vi "ClosestString.vi"(8 "array of frequencies":dbl[](array[numeric]), 11 "Detected frequency":dbl=320.0 format="%#_13g") -> (0 "Closest string":T1, 1 "index":i32, 3 "Closest frequecny":dbl)   [LabVIEW 2019]
uses:
  Strings.ctl
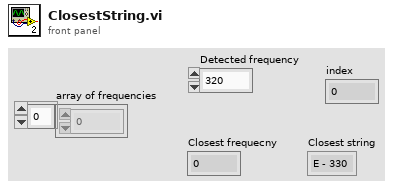
[diagram p1: front panel]
types:
  T1 = typedef "Strings.ctl" = enum16{"E - 330", "H - 247", "G - 196", "D - 147", "A - 110", "E - 82"}
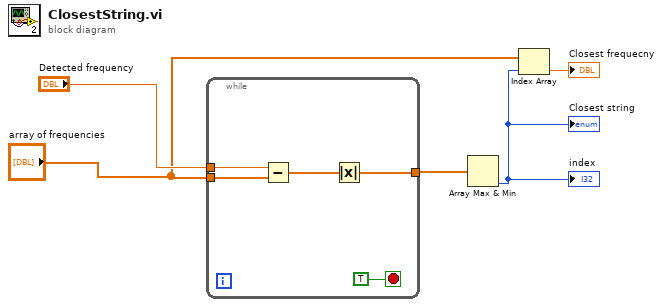
[diagram p0: block diagram]
diagram:
  n1 = while {
    tunnel: "Detected frequency" -> [w9]
    tunnel: "array of frequencies" -> [w8]
    tunnel: [w6] -> w4
    stop <- TRUE stop-if-true
    n2 = Subtract(x=w9, y=w8) -> (x-y=w7:dbl[])
    n3 = Absolute Value(x=w7) -> (abs(x)=w6:dbl[])
  }
  n4 = Array Max & Min(array=w4) -> (min index (indices)=w2:i32)  [unwired: 3 out]
  "Closest string" <- w2
  "index" <- w2
  n5 = Index Array(array="array of frequencies", index=w2) -> (element=→"Closest frequecny":dbl)
